vi "ad start prepared scan.vi"(8 "error in (no error)":errorcluster, 11 "adh":i32) -> (0 "error out":errorcluster, 3 "function return":i32)   [LabVIEW 2021, in "libad4.lvlib"]
doc: "ad_start_prepared_scan (int32_t adh);"
uses:
  <userlib>/libad4/libad4.lvlib
  <userlib>/libad4/libad4.dll
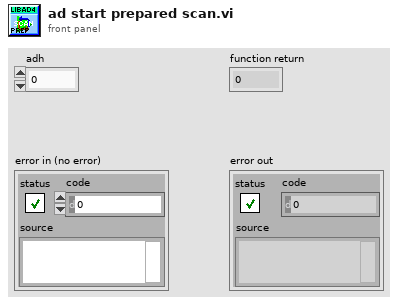
[diagram p1: front panel]
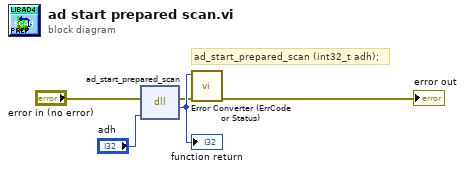
[diagram p0: block diagram]
diagram:
  # "ad_start_prepared_scan (int32_t adh);"
  n1 = dll-call lib="C:/Program Files/National Instruments/LabVIEW 2021/user.lib/libad4/libad4.*" fn="ad_start_prepared_scan"(error in="error in (no error)", "adh"="adh") -> (error out=w2:errorcluster, w5:i32)  [unwired: 3 in, 1 out]
  "function return" <- w5
  n2 = call <userlib>:"Error Converter (ErrCode or Status).vi"("error in (no error)"=w2, "error code"=w5) -> ("error out"=→"error out":errorcluster)  [unwired: 9 in]
